vi "CameraAbort.vi"(8 "error in (no error)":errorcluster, 11 "IMAQdx in":refnum<class "IMAQdx_Flea3_Firewire.lvclass">) -> (0 "error out":errorcluster, 3 "IMAQdx out":refnum<class "IMAQdx_Flea3_Firewire.lvclass">)   [LabVIEW 2012, in "IMAQdx_Flea3_Firewire.lvclass"]
uses:
  <userlib>/bias2/classes/IMAQdx_Flea3_Firewire/IMAQdx_Flea3_Firewire.lvclass
  <userlib>/bias2/classes/IMAQdx_Flea3_Firewire/IMAQdx_Flea3_Firewire.lvclass/IMAQdx_Flea3_Firewire.ctl
  <vilib>/vision/driver/NI_Vision_Acquisition_Software.lvlib
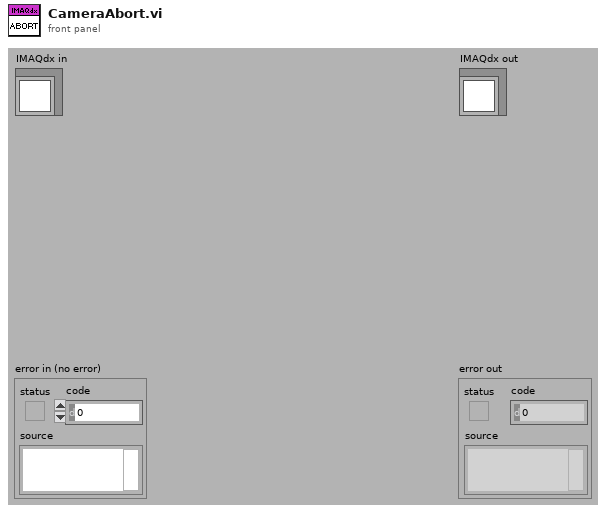
[diagram p1: front panel]
types:
  T1 = typedef "IMAQdx.ctl" = refnum<k21>
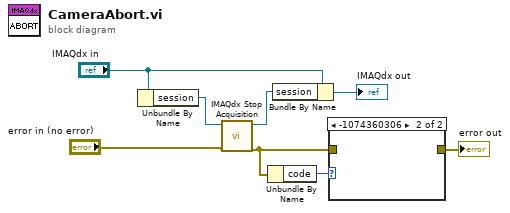
[diagram p0: block diagram]
diagram:
  n1 = Unbundle By Name("IMAQdx in") -> ("session"=w8:refnum<k21>)
  n2 = call <vilib>:"IMAQdx Stop Acquisition.vi"("error in"="error in (no error)", "Session In"=w8) -> ("error out"=w1:errorcluster, "Session Out"=w6:T1)  [unwired: 8 in]
  n3 = Unbundle By Name(w1) -> ("code"=w3:i32)
  n4 = Bundle By Name(cluster="IMAQdx in", "session"=w6) -> (→"IMAQdx out":refnum<class "IMAQdx_Flea3_Firewire.lvclass">)
  n5 = case shown="-1074360306" w3 {
    tunnel: [w9 _] -> w2
    tunnel: w1 -> [w9 _]
    frame Default {
    }
    frame -1074360306 {
    }
  }
  "error out" <- w2
